vi "FTW-JSON-Object-SetElement-null.vi"(0 "JSON":refnum<class "FTW-Container.lvclass">, 5 "Key":string, 11 "error in":errorcluster) -> (4 "JSON out":refnum<class "FTW-Container.lvclass">, 15 "error out":errorcluster)   [LabVIEW 2015]
uses:
  container/FTW-Container.lvclass
panel:
  # "Inputs"
  # "Outputs"
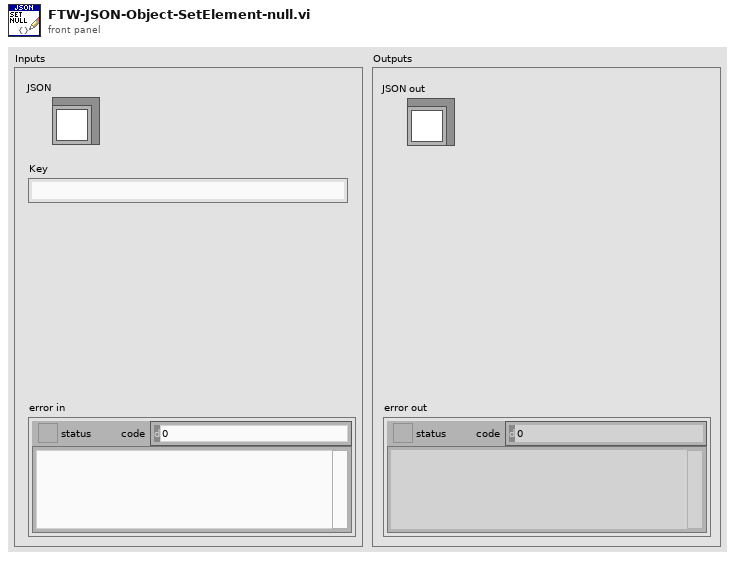
[diagram p1: front panel]
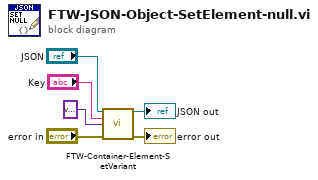
[diagram p0: block diagram]
diagram:
  n1 = call "FTW-Container-Element-SetVariant.vi"("FTW-Container In"="JSON", "Element Name"="Key", "Variant"=variant, "error in"="error in") -> ("FTW-Container Out"=→"JSON out":refnum<class "FTW-Container.lvclass">, "error out"=→"error out":errorcluster)  [unwired: 9 in, 1 out]
